vi "Configure FFT Windowing.vi"(8 "error in (no error)":errorcluster, 10 "FFT Window (0: Rectangular)":i32(ring) items=["Rectangular", "Hanning", "Flat Top", "Blackman-Harris"], 11 "VISA resource name":refnum<visa-resource-name>) -> (0 "error out":errorcluster, 3 "VISA resource name out":refnum<visa-resource-name>)   [LabVIEW 2015, in "Agilent 2000 3000 X-Series.lvlib"]
doc: "Allows the selection of four different windowing transforms or operations for the FFT (Fast Fourier Transform) function.\n\nNotes:\nOnly supported by the 3000 T Series. \nThe FFT subsystem controls the FFT function in the oscilloscope."
uses:
  <instrlib>/Agilent 2000 3000 X-Series/Agilent 2000 3000 X-Series.lvlib
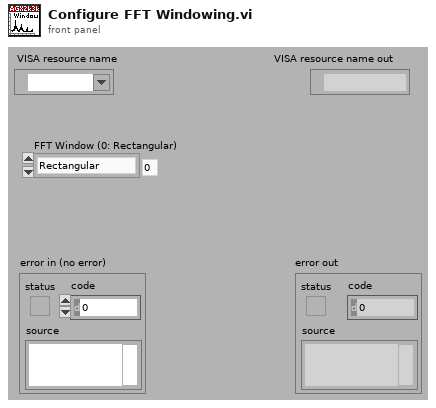
[diagram p1: front panel]
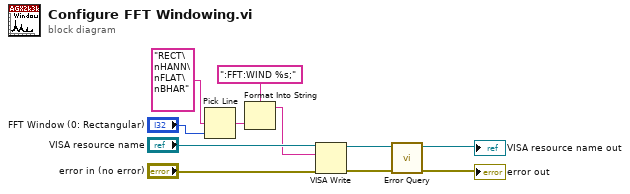
[diagram p0: block diagram]
diagram:
  n1 = Pick Line(multi-line string="RECT\nHANN\nFLAT\nBHAR", line index="FFT Window (0: Rectangular)") -> (output string=w3:string)  [unwired: 1 in]
  n2 = Format Into String(format string=":FFT:WIND %s;", w3) -> (resulting string=w6:string)  [unwired: 2 in, 1 out]
  n3 = VISA Write(VISA resource name="VISA resource name", write buffer=w6, error in (no error)="error in (no error)") -> (VISA resource name out=w10:refnum<visa-resource-name>, error out=w9:errorcluster)  [unwired: 1 out]
  n4 = call <instrlib>:"Error Query.vi"("error in (no error)"=w9, "VISA resource name"=w10) -> ("error out"=→"error out":errorcluster, "VISA resource name out"=→"VISA resource name out":refnum<visa-resource-name>)  [unwired: 8 out]
